vi "ADAM6018.vi"(4 "Scan Period":dbl format="%.2f", 5 "Previous Scan Value":dbl format="%.2f", 6 "Present scan array":dbl[](array[numeric]) format="%.2f", 7 "Value to Output":dbl format="%.2f", 8 "Ch Description":T1={"Ch Name"="", "Type"="", "Function"=enum."Analogue Input", "Ch State"=enum."On", "Calibration type"=enum."Raw", "A"=0.0, "B"=0.0, "C"=0.0, "D"=0.0, "Comments"="", "Address"={"Main"=0, "Ch."=0, "Sub"=0, "Port Name"="192.168.120.110"}, "String"="", "Duty"=65535} {"Duty" format="%.0b"; "D" format="%#_5g"; "C" format="%#_5g"; "B" format="%#_5g"; "A" format="%#_5g"}, 9 "Ch names":string[](array[string])) -> (0 "Scan comment":string, 1 "Output":dbl format="%.3f")   [LabVIEW 2014]
uses:
  ADAM Client/Sub VIs/ADAM Controls/Ch_description_ADAM.ctl
  ADAM Client/Sub VIs/ADAM Controls/Module_type_ADAM.ctl
  ADAM Client/Sub VIs/ADAM Controls/Function_ADAM.ctl
  ADAM Client/Sub VIs/ADAM Controls/Channel_State.ctl
  ADAM Client/Sub VIs/ADAM Controls/Calib_type_ADAM.ctl
  ADAM Client/Sub VIs/ADAM Controls/Address.ctl
  ADAM Serial/Serial Link Layer/NI_Modbus_Cleaned/NI Modbus121Clean.llb/MB Modbus Command.ctl
  <vilib>/Utility/error.llb/DialogType.ctl
panel:
  out "Port Name":string="192.168.120.110"
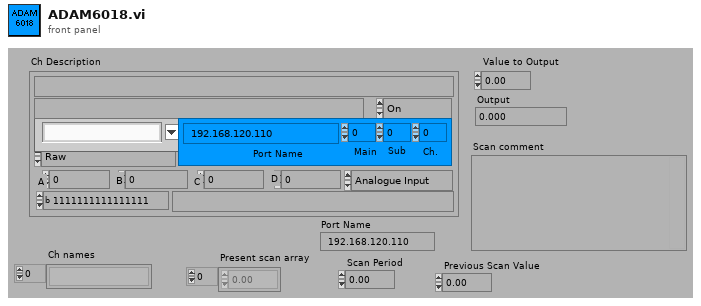
[diagram p1: front panel]
types:
  T1 = typedef "Ch_description_ADAM.ctl" = cluster{"Ch Name":string, "Type":T2, "Function":T3, "Ch State":T4, "Calibration type":T5, "A":dbl, "B":dbl, "C":dbl, "D":dbl, "Comments":string, "Address":T6, "String":string, "Duty":u16}
  T2 = typedef "Module_type_ADAM.ctl" = string
  T3 = typedef "Function_ADAM.ctl" = enum16{"Analogue Input", "Digital Input", "Event counter", "Event rate", "Analogue Output", "Digital Output", "Relay Output"}
  T4 = typedef "Channel_State.ctl" = enum16{"On", "Off", "Always On", "Always Off"}
  T5 = typedef "Calib_type_ADAM.ctl" = enum16{"Raw", "Bx + A", "Cx^2 + Bx + A", "Dx^3 + Cx^2 + Bx + A", "In Band", "Hi-Tec Q", "Hi-Tec M_dot", "Text"}
  T6 = typedef "Address.ctl" = cluster{"Main":i32, "Ch.":i32, "Sub":i32, "Port Name":string}
  T7 = typedef "DialogType.ctl" = u16
  T8 = typedef "MB Modbus Command.ctl" = cluster{"Function Code":u8, "Starting Address":u16, "Quantity":u16, "Data":u16[], "Discrete":bool[]}
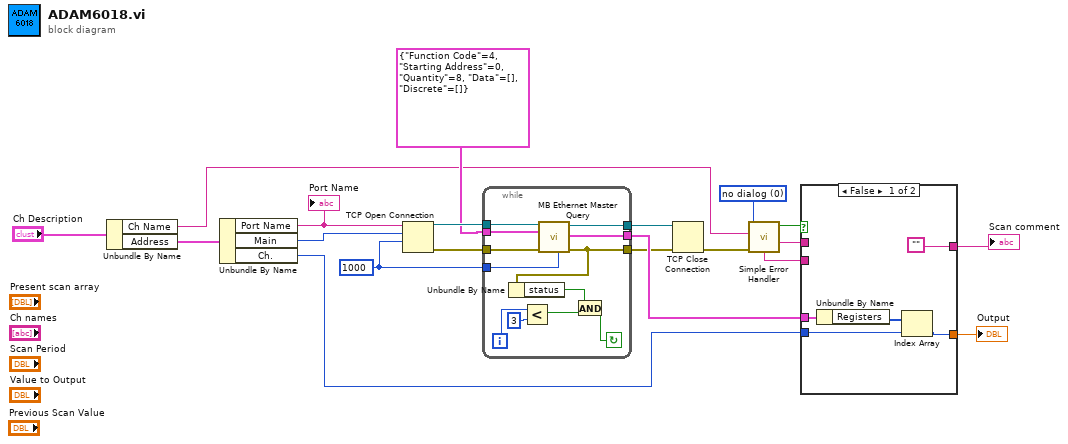
[diagram p0: block diagram]
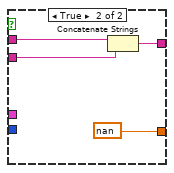
[diagram p2: hidden frame]
diagram:
  w14 = T7 0 items=["no dialog", "OK message", "continue or stop message", "OK message + warnings", "continue/stop + warnings"] ("type of dialog (OK msg:1)")
  w12 = 1000 ("Timeout")
  n1 = Unbundle By Name("Ch Description") -> ("Ch Name"=w4:string, "Address"=w6:T6)
  n2 = Unbundle By Name(w6) -> ("Port Name"=w8:string, "Main"=w7:i32, "Ch."=w5:i32)
  "Port Name" <- w8
  n3 = TCP Open Connection(address=w8, remote port or service name=w7, timeout ms (60000)=w12) -> (connection ID=w18:refnum<k5>, error out=w19:errorcluster)  [unwired: 1 in, 1 out]
  n4 = while {
    tunnel: w19 -> [w32]
    tunnel: T8 {"Function Code"=4, "Starting Address"=0, "Quantity"=8, "Data"=[], "Discrete"=[]} ("Modbus Command") -> [w30]
    tunnel: [w28] -> w16
    tunnel: w12 -> [w27]
    tunnel: [w26] -> w10
    tunnel: w18 -> [w31]
    tunnel: [w29] -> w17
    i -> [w24]
    stop <- w25 continue-if-true
    n5 = Less?(x=w24, y=3) -> (x < y?=w22:bool)
    n6 = call "MB Ethernet Master Query.vi"("Timeout"=w27, "error in (no error)"=w32, "Modbus Command"=w30, "TCP Connection Refnum in"=w31) -> ("error out"=w26:errorcluster, "Registers"=w28:cluster{"Registers":u16[], "Discrete":bool[]}, "TCP Connection Refnum (dup)"=w29:refnum<k5>)  [unwired: 3 in, 2 out]
    n7 = Unbundle By Name(w26) -> ("status"=w21:bool)
    n8 = And(x=w21, y=w22) -> (x .and. y?=w25:bool)
  }
  n9 = TCP Close Connection(connection ID=w17, error in (no error)=w10) -> (error out=w20:errorcluster)  [unwired: 2 out]
  n10 = call <vilib>:"Simple Error Handler.vi"("error source (\" \")"=w4, "type of dialog (OK msg:1)"=w14, "error in (no error)"=w20) -> ("error?"=w3:bool, "source out"=w11:string, "message"=w13:string)  [unwired: 4 out]
  n11 = case shown="False" w3 {
    tunnel: w16 -> [w37 _]
    tunnel: w13 -> [_ w39]
    tunnel: w11 -> [_ w40]
    tunnel: w5 -> [w35 _]
    tunnel: ["" w38] -> w2
    tunnel: [w34 nan ("t")] -> w1
    frame False {
      n12 = Unbundle By Name(w37) -> ("Registers"=w36:u16[])
      n13 = Index Array(array=w36, index=w35) -> (element=w34:u16)
    }
    frame True {
      n14 = Concatenate Strings(w40, w39) -> (w38:string)
    }
  }
  "Output" <- w1
  "Scan comment" <- w2
